vi "Perform measurements.vi"(6 "measurement configuration":T4={"Input channel"=0, "Full scale range"=10.0, "Input signal"=0, "Analog source resource name"="", "Sine frequency"=1000.0, "Sine amplitude"=5.1, "Triangle frequency"=20.0, "Triangle amplitude"=5.1, "Ramp duration"=10.0, "Ramp amplitude"=5.05, "Ramp type"=0, "Digital capture resource name"="", "Digital capture sample rate"=800000.0, "Digital capture test duration"=10.0} {"Ramp type" items=["Ascending", "Descending"]; "Input signal" items=["Sine", "Triangle", "Ramp"]}, 10 "meas logic calculated values":T2, 11 "measurement context in":refnum<class "MeasurementContext.lvclass">) -> (0 "error out":errorcluster, 2 "measurement results":T3)   [LabVIEW 2021, in "adc_linearityMeasurement.lvlib"]
uses:
  adc_linearityMeasurement.lvlib
  Measurement Configuration.ctl
  Measurement Results.ctl
  <vilib>/MeasurementLink/MeasurementLink Measurement Server/Classes/MeasurementContext/MeasurementContext.lvclass
  <vilib>/gRPC/LabVIEW gRPC Library/Shared/grpcId.ctl
  <vilib>/MeasurementLink/MeasurementLink Measurement Server/Classes/MeasurementContext/Accessor/Is Canceled.vi
  shared/digitalInterface/client/dcvmDPI_AD7606B_clientImpl/dcvmDPI_AD7606B_clientImpl.lvlib
  <vilib>/gRPC/LabVIEW gRPC Library/grpc-lvsupport-release.lvlib
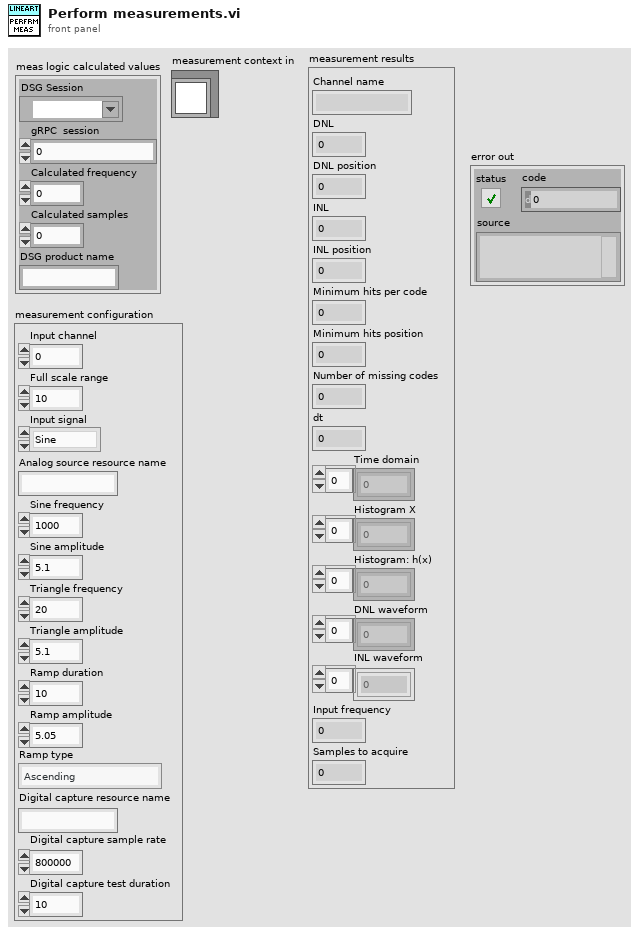
[diagram p1: front panel]
types:
  T1 = typedef "grpc-lvsupport-release.lvlib/grpcId.ctl" = u64
  T2 = cluster{"DSG Session":refnum<k21>, "gRPC  session":T1, "Calculated frequency":dbl, "Calculated samples":u32, "DSG product name":string}
  T3 = typedef "adc_linearityMeasurement.lvlib/Measurement Results.ctl" = cluster{"Channel name":string, "DNL":dbl, "DNL position":i32, "INL":dbl, "INL position":i32, "Minimum hits per code":i32, "Minimum hits position":i32, "Number of missing codes":i32, "dt":dbl, "Time domain":dbl[], "Histogram X":dbl[], "Histogram: h(x)":i32[], "DNL waveform":dbl[], "INL waveform":dbl[], "Input frequency":dbl, "Samples to acquire":u32}
  T4 = typedef "adc_linearityMeasurement.lvlib/Measurement Configuration.ctl" = cluster{"Input channel":i32, "Full scale range":dbl, "Input signal":u16, "Analog source resource name":string, "Sine frequency":dbl, "Sine amplitude":dbl, "Triangle frequency":dbl, "Triangle amplitude":dbl, "Ramp duration":dbl, "Ramp amplitude":dbl, "Ramp type":u16, "Digital capture resource name":string, "Digital capture sample rate":dbl, "Digital capture test duration":dbl}
  T5 = cluster{"X Values":dbl[], "Histogram: h(x)":i32[]}
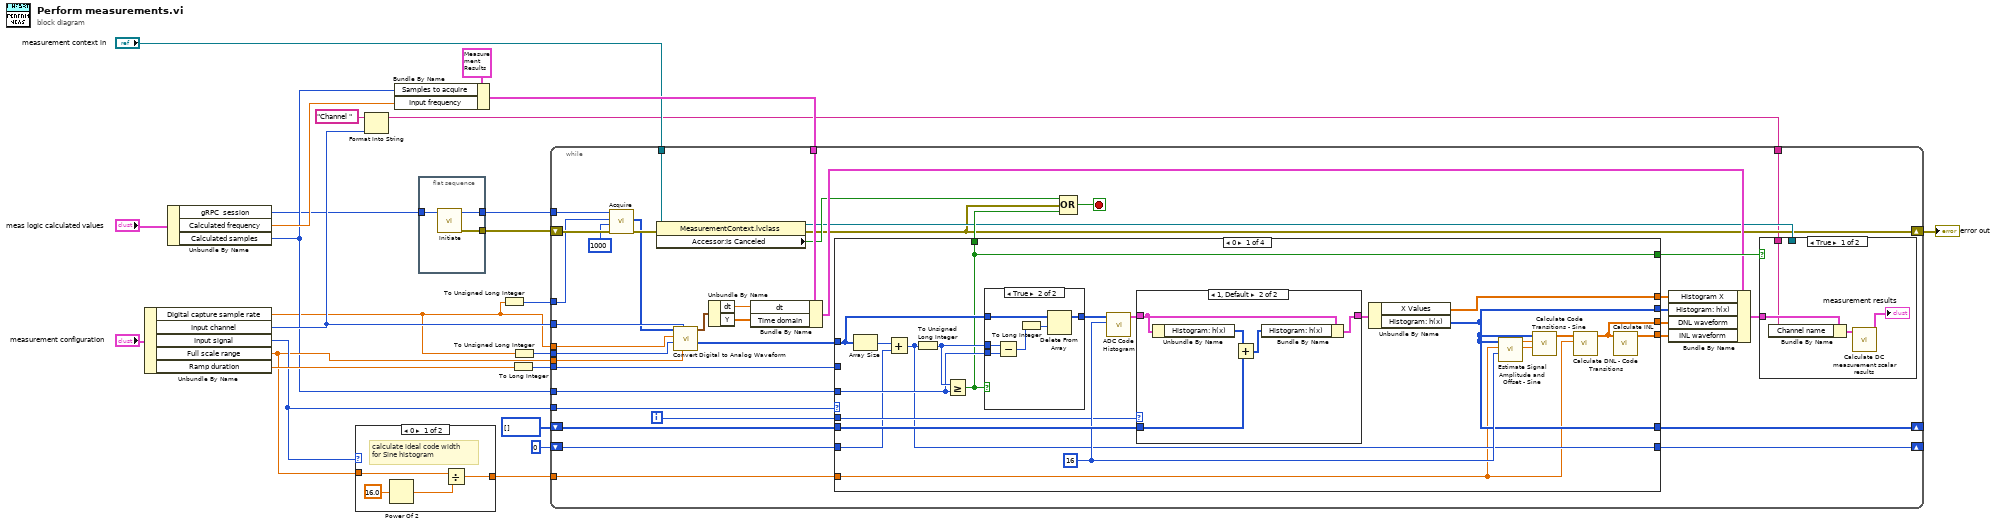
[diagram p0: block diagram]
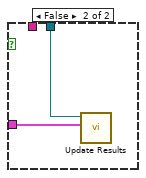
[diagram p3: hidden frame]
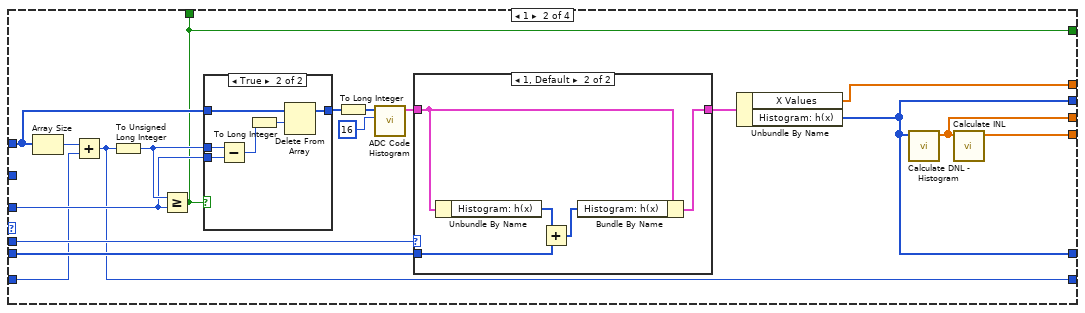
[diagram p6: hidden frame]
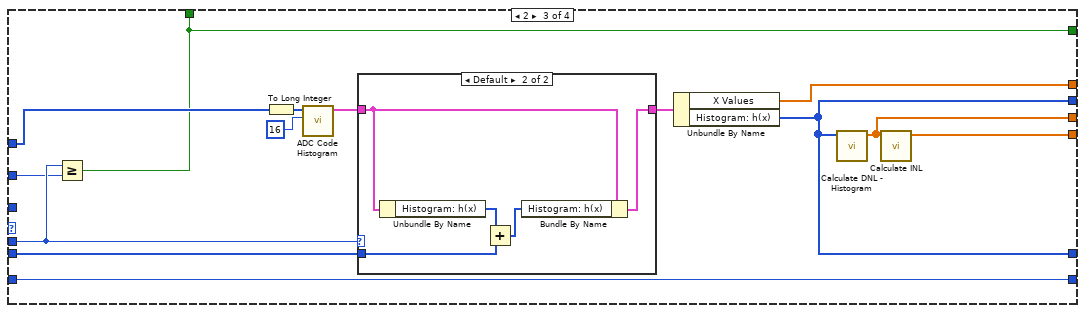
[diagram p9: hidden frame]
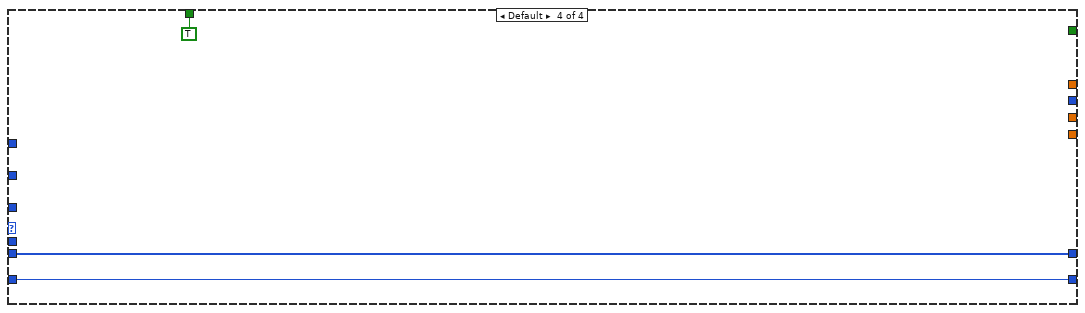
[diagram p11: hidden frame]
diagram:
  n1 = Unbundle By Name("measurement configuration") -> ("Digital capture sample rate"=w1:dbl, "Input channel"=w13:i32, "Input signal"=w17:u16, "Full scale range"=w15:dbl, "Ramp duration"=w19:dbl)
  n2 = Unbundle By Name("meas logic calculated values") -> ("gRPC  session"=w5:T1, "Calculated frequency"=w10:dbl, "Calculated samples"=w9:u32)
  n3 = case shown="0" w17 {
    tunnel: [w26 _] -> w16
    tunnel: w15 -> [w25 _]
    frame 0 {
      # "calculate ideal code width\nfor Sine histogram"
      n4 = Power Of 2(x=16.0) -> (2^x=w28:dbl)
      n5 = Divide(x=w25, y=w28) -> (x/y=w26:dbl)
    }
    frame 1, Default {
    }
  }
  n6 = Format Into String(initial string="Channel ", w13) -> (resulting string=w7:string)  [unwired: 2 in, 1 out]
  n7 = Bundle By Name(cluster=T3 {"Channel name"="", "DNL"=0.0, "DNL position"=0, "INL"=0.0, "INL position"=0, "Minimum hits per code"=0, "Minimum hits position"=0, "Number of missing codes"=0, "dt"=0.0, "Time domain"=[], "Histogram X"=[], "Histogram: h(x)"=[], "DNL waveform"=[], "INL waveform"=[], "Input frequency"=0.0, "Samples to acquire"=0} ("DC measurement results"), "Samples to acquire"=w9, "Input frequency"=w10) -> (w11:T3)
  n8 = flat-sequence {
    tunnel: w5 -> [w31]
    tunnel: [w30] -> w4
    tunnel: [w29] -> w3
    frame #0 {
      n9 = call "Initiate.vi"("gRPC session in"=w31) -> ("error out"=w29:errorcluster, "gRPC session out"=w30:T1)  [unwired: 9 in]
    }
  }
  n10 = To Unsigned Long Integer(number=w1) -> (unsigned 32bit integer=w2:u32)
  n11 = To Long Integer(number=w19) -> (32bit integer=w18:i32)
  n12 = To Unsigned Long Integer(number=w1) -> (unsigned 32bit integer=w20:u32)
  n13 = while {
    tunnel: w2 -> [w35]
    shift-right: [w39] -> w24
    shift-left: w3 -> [w36]
    tunnel: w1 -> [w69]
    tunnel: w20 -> [w68]
    tunnel: w9 -> [w66]
    shift-right: [w64] -> _
    shift-left: i32[] [] -> [w65]
    tunnel: w17 -> [w61]
    shift-right: [w58] -> _
    shift-left: 0 -> [w59]
    tunnel: w18 -> [w56]
    tunnel: w13 -> [w47]
    tunnel: w15 -> [w46]
    tunnel: w16 -> [w45]
    tunnel: w11 -> [w43]
    tunnel: "measurement context in" -> [w42]
    tunnel: w7 -> [w38]
    tunnel: w4 -> [w37]
    i -> [w60]
    stop <- w62 stop-if-true
    n14 = call "Acquire.vi"("error in"=w36, "Timeout (ms)"=1000, "Digital capture samples"=w35, "gRPC session in"=w37) -> ("error out"=w33:errorcluster, "Digital waveform"=w32:u32[])  [unwired: 5 in, 1 out]
    n15 = property class="MeasurementContext.lvclass"(reference=w42, error in=w33) -> (reference out=w40:refnum<class "MeasurementContext.lvclass">, error out=w39:errorcluster, "Accessor:Is Canceled"=w41:bool)
    n16 = call "Convert Digital to Analog Waveform.vi"("full scale range"=w46, "channel index"=w47, "Number of samples"=w68, "Sample rate"=w69, "Digital waveform in"=w32) -> ("codes"=w67:u32[], "Waveform"=w55:waveform(dbl))  [unwired: 4 in, 1 out]
    n17 = Unbundle By Name(w55) -> ("dt"=w53:dbl, "Y"=w54:dbl[])
    n18 = Bundle By Name(cluster=w43, "dt"=w53, "Time domain"=w54) -> (w52:T3)
    n19 = case shown="0" w61 {
      tunnel: w67 -> [w95 w126 w154 _]
      tunnel: w66 -> [w93 w124 _ _]
      tunnel: w65 -> [w90 w121 w152 w163]
      tunnel: [w77 w110 w141 w163] -> w64
      tunnel: [w82 w115 w147 TRUE] -> w63
      tunnel: w60 -> [w85 w119 w148 _]
      tunnel: w59 -> [w84 w117 w149 w162]
      tunnel: [w83 w116 w149 w162] -> w58
      tunnel: [w82 w115 w147 _] -> w57
      tunnel: w56 -> [_ _ w146 _]
      tunnel: [w81 w114 w145 _] -> w48
      tunnel: [w80 w113 w144 _] -> w49
      tunnel: [w77 w110 w141 _] -> w50
      tunnel: [w78 w111 w142 _] -> w51
      tunnel: w45 -> [w76 _ _ _]
      frame 0 {
        w88 = 16 ("number of bits")
        n20 = Array Size(array=w95) -> (size(s)=w96:i32)
        n21 = Add(x=w96, y=w84) -> (x+y=w83:i32)
        n22 = To Unsigned Long Integer(number=w83) -> (unsigned 32bit integer=w94:u32)
        n23 = Greater Or Equal?(x=w94, y=w93) -> (x >= y?=w82:bool)
        n24 = case shown="True" w82 {
          tunnel: w95 -> [w103 w109]
          tunnel: w94 -> [_ w108]
          tunnel: w93 -> [_ w107]
          tunnel: [w103 w104] -> w92
          frame False {
          }
          frame True {
            n25 = Subtract(x=w108, y=w107) -> (x-y=w106:u32)
            n26 = To Long Integer(number=w106) -> (32bit integer=w105:i32)
            n27 = Delete From Array(array=w109, length=w105) -> (array with subset deleted=w104:u32[])  [unwired: 1 in, 1 out]
          }
        }
        n28 = call "ADC Code Histogram.vi"("number of bits"=w88, "codes"=w92) -> ("histogram"=w91:T5)  [unwired: 8 in, 1 out]
        n29 = case shown="1, Default" w85 {
          tunnel: w91 -> [w97 w102]
          tunnel: w90 -> [_ w99]
          tunnel: [w97 w98] -> w79
          frame 0 {
          }
          frame 1, Default {
            n30 = Unbundle By Name(w102) -> ("Histogram: h(x)"=w101:i32[])
            n31 = Add(x=w101, y=w99) -> (x+y=w100:i32[])
            n32 = Bundle By Name(cluster=w102, "Histogram: h(x)"=w100) -> (w98:T5)
          }
        }
        n33 = Unbundle By Name(w79) -> ("X Values"=w78:dbl[], "Histogram: h(x)"=w77:i32[])
        n34 = call "Estimate Signal Amplitude and Offset - Sine.vi"("number of bits"=w88, "ideal code width"=w76, "histogram"=w77) -> ("estimated offset"=w86:dbl, "estimated amplitude (pk-pk)"=w87:dbl)  [unwired: 7 in]
        n35 = call "Calculate Code Transitions - Sine.vi"("midpoint offset"=w86, "estimated amplitude (pk-pk)"=w87, "histogram"=w77) -> ("code transitions"=w89:dbl[])  [unwired: 7 in, 1 out]
        n36 = call "Calculate DNL - Code Transitions.vi"("ideal code width"=w76, "code transitions"=w89) -> ("DNL"=w80:dbl[])  [unwired: 9 in]
        n37 = call "Calculate INL.vi"("DNL"=w80) -> ("INL"=w81:dbl[])  [unwired: 10 in]
      }
      frame 1 {
        n38 = Array Size(array=w126) -> (size(s)=w127:i32)
        n39 = Add(x=w127, y=w117) -> (x+y=w116:i32)
        n40 = To Unsigned Long Integer(number=w116) -> (unsigned 32bit integer=w125:u32)
        n41 = Greater Or Equal?(x=w125, y=w124) -> (x >= y?=w115:bool)
        n42 = case shown="True" w115 {
          tunnel: w126 -> [w134 w140]
          tunnel: w125 -> [_ w139]
          tunnel: w124 -> [_ w138]
          tunnel: [w134 w135] -> w123
          frame False {
          }
          frame True {
            n43 = Subtract(x=w139, y=w138) -> (x-y=w137:u32)
            n44 = To Long Integer(number=w137) -> (32bit integer=w136:i32)
            n45 = Delete From Array(array=w140, length=w136) -> (array with subset deleted=w135:u32[])  [unwired: 1 in, 1 out]
          }
        }
        n46 = To Long Integer(number=w123) -> (32bit integer=w118:i32[])
        n47 = call "ADC Code Histogram.vi"("number of bits"=16, "codes"=w118) -> ("histogram"=w122:T5)  [unwired: 8 in, 1 out]
        n48 = case shown="1, Default" w119 {
          tunnel: w122 -> [w128 w133]
          tunnel: w121 -> [_ w130]
          tunnel: [w128 w129] -> w112
          frame 0 {
          }
          frame 1, Default {
            n49 = Unbundle By Name(w133) -> ("Histogram: h(x)"=w132:i32[])
            n50 = Add(x=w132, y=w130) -> (x+y=w131:i32[])
            n51 = Bundle By Name(cluster=w133, "Histogram: h(x)"=w131) -> (w129:T5)
          }
        }
        n52 = Unbundle By Name(w112) -> ("X Values"=w111:dbl[], "Histogram: h(x)"=w110:i32[])
        n53 = call "Calculate DNL - Histogram.vi"("histogram"=w110) -> ("DNL"=w113:dbl[])  [unwired: 10 in]
        n54 = call "Calculate INL.vi"("DNL"=w113) -> ("INL"=w114:dbl[])  [unwired: 10 in]
      }
      frame 2 {
        n55 = Greater Or Equal?(x=w148, y=w146) -> (x >= y?=w147:bool)
        n56 = To Long Integer(number=w154) -> (32bit integer=w150:i32[])
        n57 = call "ADC Code Histogram.vi"("number of bits"=16, "codes"=w150) -> ("histogram"=w153:T5)  [unwired: 8 in, 1 out]
        n58 = case shown="Default" w148 {
          tunnel: w153 -> [w155 w160]
          tunnel: w152 -> [_ w157]
          tunnel: [w155 w156] -> w143
          frame 0 {
          }
          frame Default {
            n59 = Unbundle By Name(w160) -> ("Histogram: h(x)"=w159:i32[])
            n60 = Add(x=w159, y=w157) -> (x+y=w158:i32[])
            n61 = Bundle By Name(cluster=w160, "Histogram: h(x)"=w158) -> (w156:T5)
          }
        }
        n62 = Unbundle By Name(w143) -> ("X Values"=w142:dbl[], "Histogram: h(x)"=w141:i32[])
        n63 = call "Calculate DNL - Histogram.vi"("histogram"=w141) -> ("DNL"=w144:dbl[])  [unwired: 10 in]
        n64 = call "Calculate INL.vi"("DNL"=w144) -> ("INL"=w145:dbl[])  [unwired: 10 in]
      }
      frame Default {
      }
    }
    n65 = Compound Arithmetic op=OR(w41, w39, w63) -> (w62:bool)
    n66 = Bundle By Name(cluster=w52, "Histogram X"=w51, "Histogram: h(x)"=w50, "DNL waveform"=w49, "INL waveform"=w48) -> (w44:T3)
    n67 = case shown="True" w57 {
      tunnel: w40 -> [_ w75]
      tunnel: w44 -> [w72 w74]
      tunnel: w38 -> [w71 _]
      frame True {
        n68 = Bundle By Name(cluster=w72, "Channel name"=w71) -> (w70:T3)
        n69 = call "Calculate DC measurement scalar results.vi"("DC measurement results"=w70) -> ("output cluster"=→"measurement results":T3)  [unwired: 10 in]
      }
      frame False {
        n70 = call <vilib>:"Update Results.vi"("Measurement Results"=w74, "MeasurementContext in"=w75) -> ()  [unwired: 8 in, 2 out]
      }
    }
  }
  "error out" <- w24
